vi "sub vi - AI USB4704 (3) v73.vi"(0 "Task0":i32, 5 "Task1":i32, 7 "Task2":i32, 11 "SAMPLES":dbl) -> (4 "data 0":waveform(dbl)[](array[waveform]), 6 "data 1":waveform(dbl)[](array[waveform]), 8 "data 2":waveform(dbl)[](array[waveform]), 10 "loop time":dbl format="%.6g", 15 "error array":errorcluster[](array[cluster]))   [LabVIEW 2017]
uses:
  <userlib>/DAQNavi Polymorphic VI/read/DAQNavi Read (Analog 1D Wfm NChan NSamp).vi
panel:
  out "Fault 3":bool
  out "Fault 2":bool
  out "Fault 1":bool
  out "String":string
  in  "Tab Control":enum32{"USB #0", "USB #1", "USB #2"}(tab)
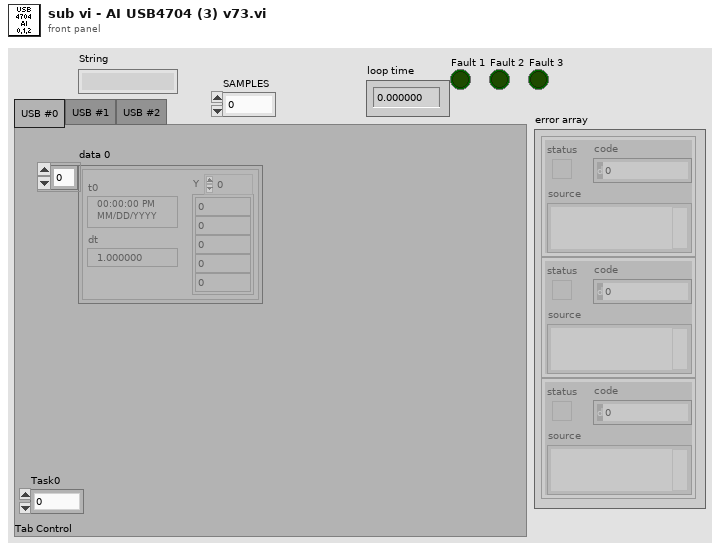
[diagram p1: front panel]
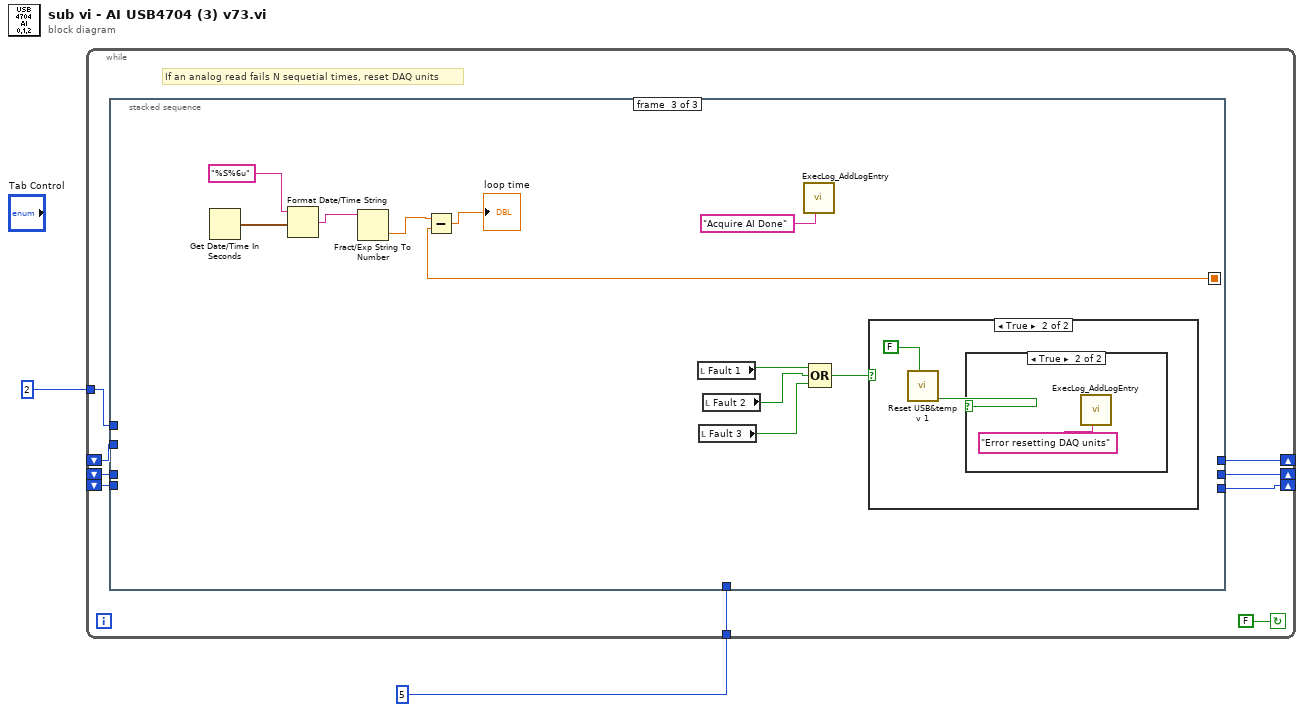
[diagram p0: block diagram]
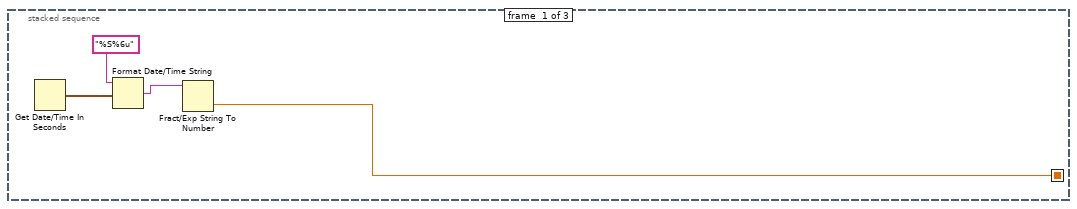
[diagram p2: hidden frame]
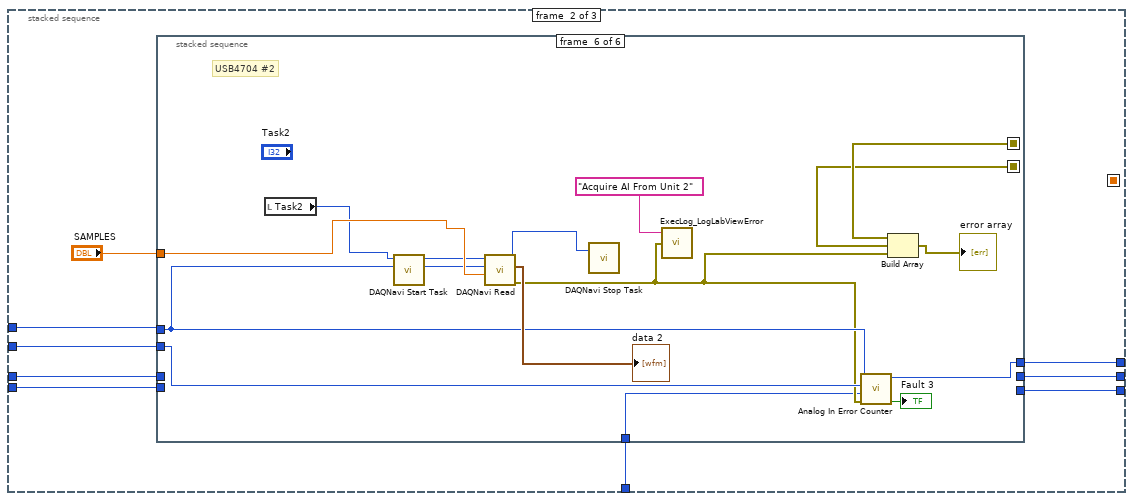
[diagram p3: hidden frame]
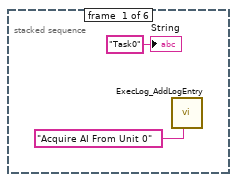
[diagram p4: hidden frame]
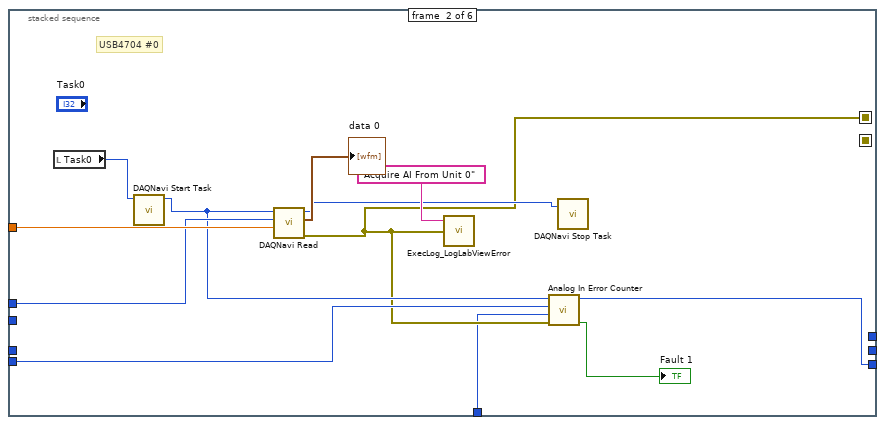
[diagram p5: hidden frame]
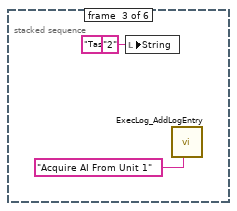
[diagram p6: hidden frame]
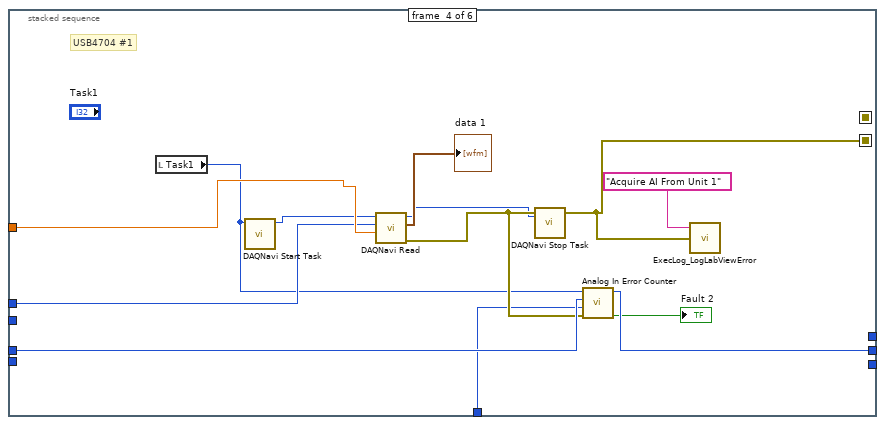
[diagram p7: hidden frame]
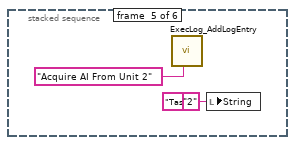
[diagram p8: hidden frame]
diagram:
  n1 = while {
    tunnel: 2 -> [w11]
    shift-right: [w10] -> _
    shift-left: _ -> [w9]
    shift-right: [w7] -> _
    shift-left: _ -> [w8]
    shift-right: [w5] -> _
    shift-left: _ -> [w6]
    tunnel: 5 ("Max Errors") -> [w3]
    stop <- FALSE continue-if-true
    # "If an analog read fails N sequetial times, reset DAQ units"
    n2 = stacked-sequence {
      seq-local: [w12 _ _] -> [_ _ w78]
      tunnel: w11 -> [_ w24 _]
      tunnel: [_ w22 _] -> w10
      tunnel: w9 -> [_ w21 _]
      tunnel: w8 -> [_ w20 _]
      tunnel: [_ w19 _] -> w7
      tunnel: w6 -> [_ w18 _]
      tunnel: [_ w17 _] -> w5
      tunnel: w3 -> [_ w16 _]
      frame #0 {
        n3 = Get Date/Time In Seconds() -> (seconds since 1Jan1904=w14:timestamp)
        n4 = Format Date/Time String(time format string (%c)="%S%6u", seconds (now)=w14) -> (date/time string=w13:string)  [unwired: 1 in]
        n5 = Fract/Exp String To Number(string=w13) -> (number=w12:dbl)  [unwired: 3 in, 1 out]
      }
      frame #1 {
        n6 = stacked-sequence {
          seq-local: [_ w29 _ _ _ _] -> [_ _ _ _ _ w70]
          seq-local: [_ _ _ w46 _ _] -> [_ _ _ _ _ w69]
          tunnel: "SAMPLES" -> [_ w38 _ w53 _ w71]
          tunnel: w24 -> [_ w37 _ w52 _ w64]
          tunnel: [_ _ _ _ _ w65] -> w22
          tunnel: w21 -> [_ _ _ _ _ w66]
          tunnel: w20 -> [_ _ _ w50 _ _]
          tunnel: [_ _ _ w49 _ _] -> w19
          tunnel: w18 -> [_ w35 _ _ _ _]
          tunnel: [_ w34 _ _ _ _] -> w17
          tunnel: w16 -> [_ w28 _ w42 _ w57]
          frame #0 {
            n7 = call "ExecLog_AddLogEntry.vi"("Msg"="Acquire AI From Unit 0") -> ()  [unwired: 7 in, 3 out]
            "String" <- "Task0" ("String")
          }
          frame #1 {
            # "USB4704 #0"
            n8 = local read "Task0"() -> (w32:i32)
            n9 = call <userlib>:"DAQNavi Start Task.vi"("task in"=w32) -> ("task out"=w31:i32)  [unwired: 9 in, 1 out]
            n10 = call-poly <userlib>:"DAQNavi Read.vi"("number of samples per channel to read"=w38, "timeout"=w37, "task in"=w31) -> ("error out"=w29:errorcluster, "data"=→"data 0":waveform(dbl)[], "task out"=w30:i32)  [unwired: 1 in, 5 out]
            n11 = call "ExecLog_LogLabViewError.vi"("error IO"=w29, "string 1"="Acquire AI From Unit 0" ("Msg")) -> ()  [unwired: 2 in, 1 out]
            n12 = call "Analog In Error Counter.vi"("error in (no error)"=w29, "Max Errors"=w28, "Count"=w35, "Unit"=w31) -> ("Fault"=→"Fault 1":bool, "Numeric out"=w34:i32)  [unwired: 6 in]
            n13 = call <userlib>:"DAQNavi Stop Task.vi"("task in"=w30) -> ()  [unwired: 1 in, 2 out]
          }
          frame #2 {
            n14 = local write "String"("Task1" ("String")) -> ()
            n15 = local write "String"("2" ("String")) -> ()
            n16 = call "ExecLog_AddLogEntry.vi"("Msg"="Acquire AI From Unit 1") -> ()  [unwired: 7 in, 3 out]
          }
          frame #3 {
            # "USB4704 #1"
            n17 = local read "Task1"() -> (w44:i32)
            n18 = call <userlib>:"DAQNavi Start Task.vi"("task in"=w44) -> ("task out"=w43:i32)  [unwired: 9 in, 1 out]
            n19 = call-poly <userlib>:"DAQNavi Read.vi"("number of samples per channel to read"=w53, "timeout"=w52, "task in"=w43) -> ("error out"=w46:errorcluster, "data"=→"data 1":waveform(dbl)[], "task out"=w45:i32)  [unwired: 1 in, 5 out]
            n20 = call <userlib>:"DAQNavi Stop Task.vi"("task in"=w45) -> ()  [unwired: 1 in, 2 out]
            n21 = call "Analog In Error Counter.vi"("error in (no error)"=w46, "Max Errors"=w42, "Count"=w50, "Unit"=w44) -> ("Fault"=→"Fault 2":bool, "Numeric out"=w49:i32)  [unwired: 6 in]
            n22 = call "ExecLog_LogLabViewError.vi"("error IO"=w46, "string 1"="Acquire AI From Unit 1" ("Msg")) -> ()  [unwired: 2 in, 1 out]
          }
          frame #4 {
            n23 = call "ExecLog_AddLogEntry.vi"("Msg"="Acquire AI From Unit 2") -> ()  [unwired: 7 in, 3 out]
            n24 = local write "String"("Task2" ("String")) -> ()
            n25 = local write "String"("2" ("String")) -> ()
          }
          frame #5 {
            # "USB4704 #2"
            n26 = local read "Task2"() -> (w60:i32)
            n27 = call <userlib>:"DAQNavi Start Task.vi"("task in"=w60) -> ("task out"=w59:i32)  [unwired: 9 in, 1 out]
            n28 = call-poly <userlib>:"DAQNavi Read.vi"("number of samples per channel to read"=w71, "timeout"=w64, "task in"=w59) -> ("error out"=w61:errorcluster, "data"=→"data 2":waveform(dbl)[], "task out"=w58:i32)  [unwired: 1 in, 5 out]
            n29 = call <userlib>:"DAQNavi Stop Task.vi"("task in"=w58) -> ()  [unwired: 1 in, 2 out]
            n30 = call "ExecLog_LogLabViewError.vi"("error IO"=w61, "string 1"="Acquire AI From Unit 2" ("Msg")) -> ()  [unwired: 2 in, 1 out]
            n31 = call "Analog In Error Counter.vi"("error in (no error)"=w61, "Max Errors"=w57, "Count"=w66, "Unit"=w64) -> ("Fault"=→"Fault 3":bool, "Numeric out"=w65:i32)  [unwired: 6 in]
            n32 = Build Array(w70, w69, w61) -> (→"error array":errorcluster[])
          }
        }
      }
      frame #2 {
        n33 = Get Date/Time In Seconds() -> (seconds since 1Jan1904=w81:timestamp)
        n34 = Format Date/Time String(time format string (%c)="%S%6u", seconds (now)=w81) -> (date/time string=w80:string)  [unwired: 1 in]
        n35 = Fract/Exp String To Number(string=w80) -> (number=w79:dbl)  [unwired: 3 in, 1 out]
        n36 = Subtract(x=w79, y=w78) -> (x-y=→"loop time":dbl)
        n37 = local read "Fault 1"() -> (w76:bool)
        n38 = local read "Fault 3"() -> (w74:bool)
        n39 = local read "Fault 2"() -> (w75:bool)
        n40 = call "ExecLog_AddLogEntry.vi"("Msg"="Acquire AI Done") -> ()  [unwired: 7 in, 3 out]
        n41 = Compound Arithmetic op=OR(w76, w75, w74) -> (w73:bool)
        n42 = case shown="True" w73 {
          frame False {
          }
          frame True {
            n43 = call "Reset USB&temp v 1.vi"("Test"=FALSE) -> ("Reset Error"=w83:bool)  [unwired: 10 in]
            n44 = case shown="True" w83 {
              frame False {
              }
              frame True {
                n45 = call "ExecLog_AddLogEntry.vi"("Msg"="Error resetting DAQ units" ("message")) -> ()  [unwired: 7 in, 3 out]
              }
            }
          }
        }
      }
    }
  }
